vi "ConvertData.vi"(10 "数组":string[](array[string])) -> (2 "数组 2":u16[](array[numeric]) format="%.0x")   [LabVIEW 2020]
panel:
  out "电子表格字符串":string
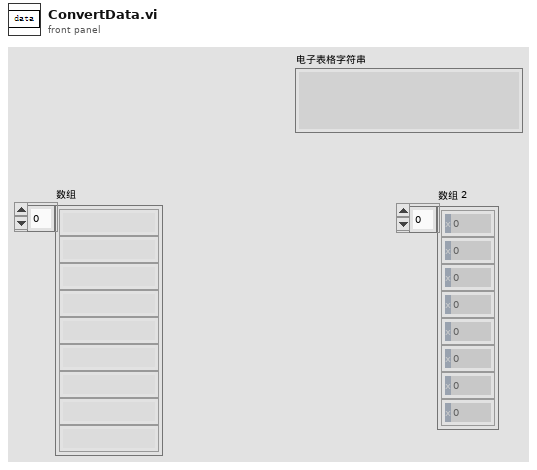
[diagram p1: front panel]
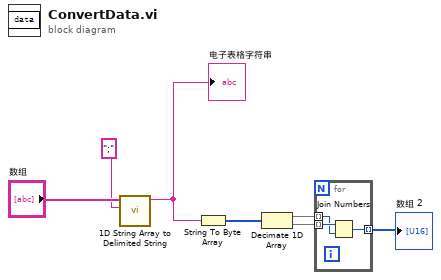
[diagram p0: block diagram]
diagram:
  n1 = call <vilib>:"1D String Array to Delimited String.vi"("delimiter"=";" ("分隔符(Tab)"), "string array"="数组") -> ("delimited string"=w1:string)  [unwired: 9 in]
  "电子表格字符串" <- w1
  n2 = String To Byte Array(string=w1) -> (unsigned byte array=w7:u8[])
  n3 = Decimate 1D Array(w7) -> (w6:u8[], w5:u8[])
  n4 = for {
    tunnel: w6 -> [w9] mode=indexing
    tunnel: w5 -> [w10] mode=indexing
    tunnel: [w8] -> w4 mode=indexing
    n5 = Join Numbers(hi=w10, lo=w9) -> ((hi.lo)=w8:u16)
  }
  "数组 2" <- w4
